vi "Lab3BoydJoya.vi"() -> ()   [LabVIEW 2011]
uses:
  <vilib>/robotics/Starter Kit/2.0/9632 Host Interface/NI_Robotics_Starter Kit Host_9632_2.0.lvclass
  <vilib>/robotics/Starter Kit/Host Interface/NI_Robotics_Starter Kit Host.lvclass
panel:
  in  "stop":bool
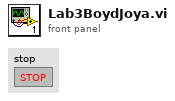
[diagram p1: front panel]
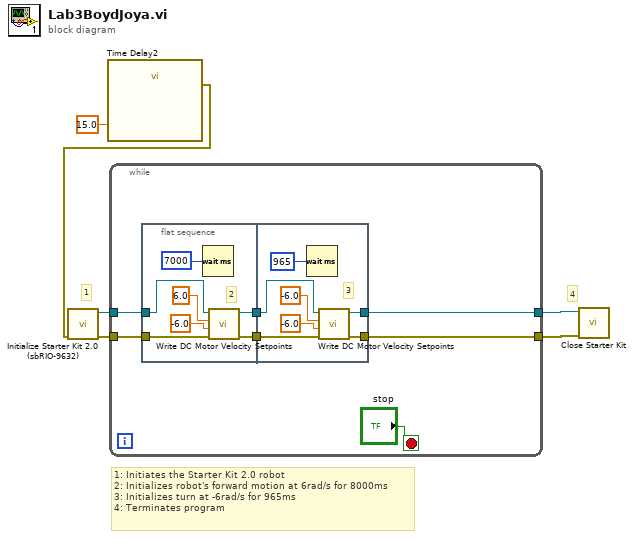
[diagram p0: block diagram]
diagram:
  # "1: Initiates the Starter Kit 2.0 robot\n2: Initializes robot's forward motion at 6rad/s for 8000ms\n3: Initializes turn at -6rad/s for 965ms\n4: Terminates program"
  # "4"
  # "1"
  n1 = call "Time Delay2"("Delay Time (s)"=15.0) -> ("error out"=w2:errorcluster)  [unwired: 10 in]
  n2 = call <vilib>:"Initialize Starter Kit 2.0 (sbRIO-9632).vi"("error in (no error)"=w2) -> ("error out"=w5:errorcluster, "FPGA starter kit host 2.0 out"=w6:refnum<class "NI_Robotics_Starter Kit Host_9632_2.0.lvclass">)  [unwired: 9 in]
  n3 = while {
    tunnel: [w11] -> w3
    tunnel: [w10] -> w4
    tunnel: w6 -> [w9]
    tunnel: w5 -> [w8]
    stop <- "stop" stop-if-true
    n4 = flat-sequence {
      tunnel: [w18] -> w13
      tunnel: [w17] -> w12
      tunnel: w9 -> [w15]
      tunnel: w8 -> [w14]
      tunnel: w13 -> [w25]
      tunnel: w12 -> [w24]
      tunnel: [w23] -> w11
      tunnel: [w22] -> w10
      frame #0 {
        # "2"
        n5 = Wait (ms)(milliseconds to wait=u32 7000) -> ()  [unwired: 1 out]
        n6 = call <vilib>:"Write DC Motor Velocity Setpoints.vi"("error in (no error)"=w14, "right motor ccw velocity (rad/s)"=-6.0, "left motor ccw velocity (rad/s)"=6.0, "starter kit host in"=w15) -> ("error out"=w17:errorcluster, "starter kit host out"=w18:refnum<class "NI_Robotics_Starter Kit Host_9632_2.0.lvclass">)  [unwired: 6 in]
      }
      frame #1 {
        # "3"
        n7 = Wait (ms)(milliseconds to wait=u32 965) -> ()  [unwired: 1 out]
        n8 = call <vilib>:"Write DC Motor Velocity Setpoints.vi"("error in (no error)"=w24, "right motor ccw velocity (rad/s)"=-6.0, "left motor ccw velocity (rad/s)"=-6.0, "starter kit host in"=w25) -> ("error out"=w22:errorcluster, "starter kit host out"=w23:refnum<class "NI_Robotics_Starter Kit Host_9632_2.0.lvclass">)  [unwired: 6 in]
      }
    }
  }
  n9 = call-dynamic "Close Starter Kit.vi"("error in (no error)"=w4, "starter kit host in"=w3) -> ()  [unwired: 9 in, 1 out]
